vi "Motor.vi"(11 "Angle (deg)":sgl) -> (3 "3D Picture Control":refnum<vi>(3d-picture))   [LabVIEW 2013]
uses:
  <vilib>/picture/3D Picture Control/NI_3D Picture Control.lvlib
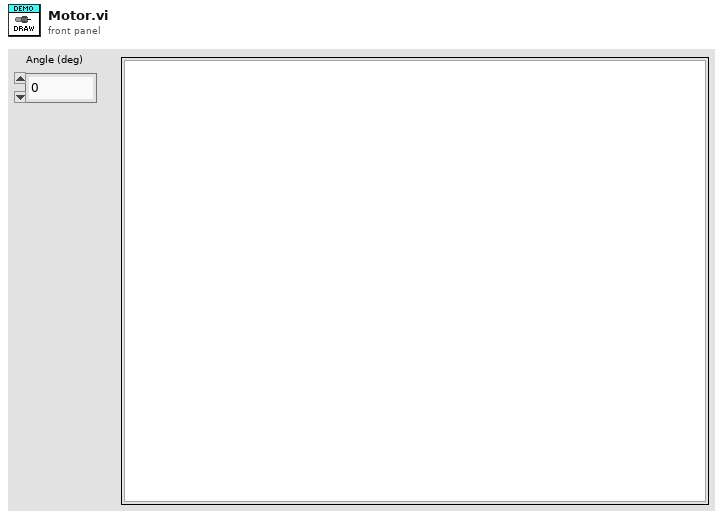
[diagram p1: front panel]
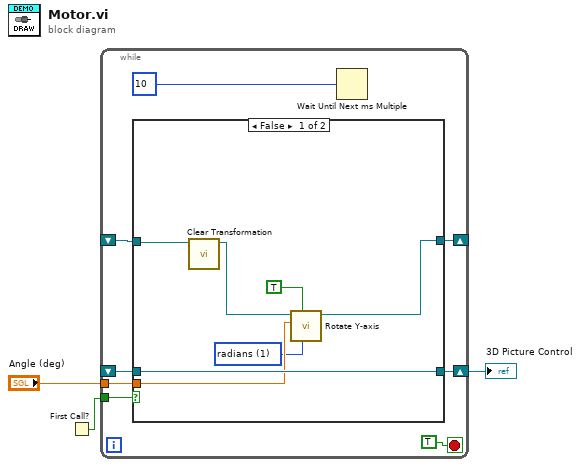
[diagram p0: block diagram]
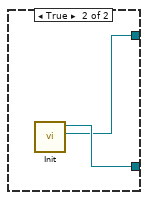
[diagram p2: hidden frame]
diagram:
  n1 = First Call?() -> (First Call?: T/F=w3:bool)
  n2 = while {
    tunnel: w3 -> [w10]
    shift-right: [w8] -> _
    shift-left: _ -> [w6]
    shift-right: [w9] -> w2
    shift-left: _ -> [w7]
    tunnel: "Angle (deg)" -> [w5]
    stop <- TRUE stop-if-true
    n3 = case shown="False" w10 {
      tunnel: [w18 w20] -> w9
      tunnel: [w16 w19] -> w8
      tunnel: w7 -> [w18 _]
      tunnel: w6 -> [w15 _]
      tunnel: w5 -> [w17 _]
      frame False {
        w12 = u16 1 items=["degree", "radians"] ("angle unit")
        n4 = call <vilib>:"Clear Transformation.vi"("Object Refnum In"=w15) -> ("Object Refnum Out"=w13:refnum<vi>)  [unwired: 9 in, 1 out]
        n5 = call <vilib>:"Rotate Y-axis.vi"("angle unit"=w12, "Relative?"=TRUE, "angle"=w17, "Scene Object In"=w13) -> ("Scene Object Out"=w16:refnum<vi>)  [unwired: 6 in, 1 out]
      }
      frame True {
        n6 = call "Init.vi"() -> ("Propeller"=w19:refnum<vi>, "Scene Object Out"=w20:refnum<vi>)  [unwired: 9 in, 1 out]
      }
    }
    n7 = Wait Until Next ms Multiple(millisecond multiple=10) -> ()  [unwired: 1 out]
  }
  "3D Picture Control" <- w2
